vi "Multiples_of_3_or_5_Template.vi"(4 "Maximum":i32) -> (0 "Sum":i32, 2 "Multiples":i32[](array[numeric]))   [LabVIEW 2013]
panel:
  # "Multiples of 3 or 5\n\nIf we list all the natural numbers below 10 that are multiples of 3 or 5, we get 3, 5, 6 and 9. \nThe sum of these multiples is 23. \n\nCreate a VI that takes one numeric input representing the maximum number and generates an \narray of all multiples of 3 or 5 that are strictly less than that number as well as the sum of all of \nthe multiples."
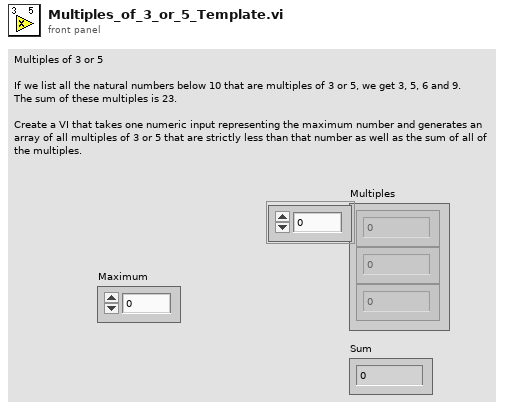
[diagram p1: front panel]
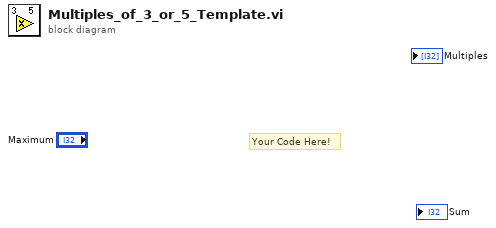
[diagram p0: block diagram]
diagram:
  # "Your Code Here!"
